vi "Test ARGB to-from Greyscale.vi"(8 "error in (no error)":errorcluster, 11 "Test Case In":refnum<class "01_Image.lvclass">) -> (0 "error out":errorcluster, 3 "Test Case Out":refnum<class "01_Image.lvclass">)   [LabVIEW 2020, in "test.lvlib" / "01_Image.lvclass"]
uses:
  01_Image.lvclass
  C:/Program Files (x86)/National Instruments/LabVIEW 2026/vi.lib/Astemes/LUnit/Test Case.lvclass
  common/Image Size (Integer).ctl
  <vilib>/Astemes/LUnit/Test Case.lvclass/Test Case.ctl
  image/New Image (Greyscale Preallocated).vi
  image/New Image (ARGB Preallocated).vi
  4993e8ee-a06a-463a-9684-69129f64d5ce.vi
  image/Copy Array to Image.vi
  image/Copy Array to Image (ARGB).vi
  image/New Image (Greyscale Preallocated).vi/6598b9e0-8a08-46f5-91fd-ca1b87217137.vi
  image/ARGBExtractChannel.vi
  image/New Image (ARGB Preallocated).vi/3321fa97-f432-4e1e-8db9-a0df79aed21b.vi
  image/ARGB Colour to U32 Pixel Value.vi
  <vilib>/Astemes/LUnit/Core/LUnit Test Case/Private/Append Pass Result.vi
  <vilib>/Astemes/LUnit/Core/LUnit Test Case/Private/Append Fail Result.vi
  4993e8ee-a06a-463a-9684-69129f64d5ce.vi/9c5d11cd-9439-4240-a1ee-d9baace9c924.vi
  <vilib>/Astemes/LUnit/Core/LUnit Test Case/Private/Run In UI.vi
  <vilib>/Utility/error.llb/Clear Errors.vi
  <vilib>/Utility/error.llb/Error Cluster From Error Code.vi
  <vilib>/picture/pixmap.llb/Flatten Pixmap.vi
  image/image.lvlib
  common/common.lvlib
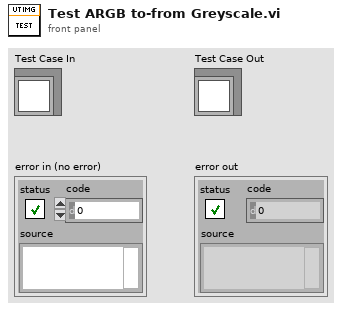
[diagram p1: front panel]
types:
  T1 = typedef "common.lvlib/Image Size (Integer).ctl" = cluster{"Width":u16, "Height":u16}
  T2 = typedef "image.lvlib/ARGB Image.ctl" = refnum<data-value>
  T3 = typedef "image.lvlib/Greyscale Image.ctl" = refnum<data-value>
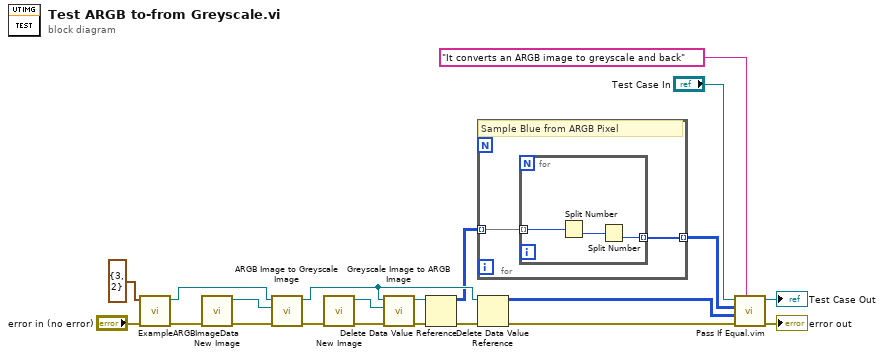
[diagram p0: block diagram]
diagram:
  n1 = call "ExampleARGBImageData.vi"("error in (no error)"="error in (no error)", "Image Size"=T1 {"Width"=3, "Height"=2}) -> ("error out"=w16:errorcluster, "Data Value Reference out"=w8:T2)  [unwired: 6 in, 2 out]
  n2 = call-poly "New Image.vi"("error in (no error)"=w16) -> ("error out"=w14:errorcluster, "Greyscale Image"=w17:T3)  [unwired: 9 in]
  n3 = call "ARGB Image to Greyscale Image.vi"("error in (no error)"=w14, "Greyscale Image Destination in"=w17, "ARGB Image Source in"=w8) -> ("error out"=w13:errorcluster, "Greyscale Image Destination"=w7:T3)  [unwired: 7 in]
  n4 = call-poly "New Image.vi"("error in (no error)"=w13) -> ("error out"=w11:errorcluster, "ARGB Image"=w12:T2)  [unwired: 9 in]
  n5 = call "Greyscale Image to ARGB Image.vi"("error in (no error)"=w11, "ARGB Image Destination in"=w12, "Greyscale Image Source in"=w7) -> ("error out"=w9:errorcluster, "ARGB Image Destination"=w10:T2)  [unwired: 7 in]
  n6 = Delete Data Value Reference(data value reference=w10, error in=w9) -> (data value=w3:u32[][], error out=w6:errorcluster)
  n7 = for {
    tunnel: w3 -> [w23] mode=indexing
    tunnel: [w22] -> w2 mode=indexing
    # "Sample Blue from ARGB Pixel"
    n8 = for {
      tunnel: w23 -> [w26] mode=indexing
      tunnel: [w24] -> w22 mode=indexing
      n9 = Split Number(x=w26) -> (lo(x)=w25:u16)  [unwired: 1 out]
      n10 = Split Number(x=w25) -> (lo(x)=w24:u8)  [unwired: 1 out]
    }
  }
  n11 = Delete Data Value Reference(data value reference=w7, error in=w6) -> (data value=w4:u8[][], error out=w5:errorcluster)
  n12 = call "Pass If Equal.vim"("Description"="It converts an ARGB image to greyscale and back", "error in (no error)"=w5, "Actual"=w4, "Expected"=w2, "LUnit Test Case In"="Test Case In") -> ("error out"=→"error out":errorcluster, "LUnit Test Case Out"=→"Test Case Out":refnum<class "01_Image.lvclass">)  [unwired: 5 in]
